vi "Execute.vi"(0 "Session Handle in":T4, 1 "Sequence Name":string, 5 "SequenceFile":T3, 9 "Parameters (None)":T2, 11 "error in (no error)":errorcluster, 12 "ProcessModel (None)":T3) -> (4 "Session Handle out":T4, 10 "Execution":T1, 15 "error out":errorcluster)   [LabVIEW 2019, in "HTS.lvlib" / "Engine.lvclass"]
uses:
  Engine.lvclass
  Typedefs/Session Handle.ctl
  SequenceFile/SequenceFile.lvclass
  SequenceFile/Typedefs/Session Handle.ctl
  VariableContainer/VariableContainer.lvclass
  VariableContainer/Typedefs/Session Handle.ctl
  Execution/Execution.lvclass
  Execution/Typedefs/Session Handle.ctl
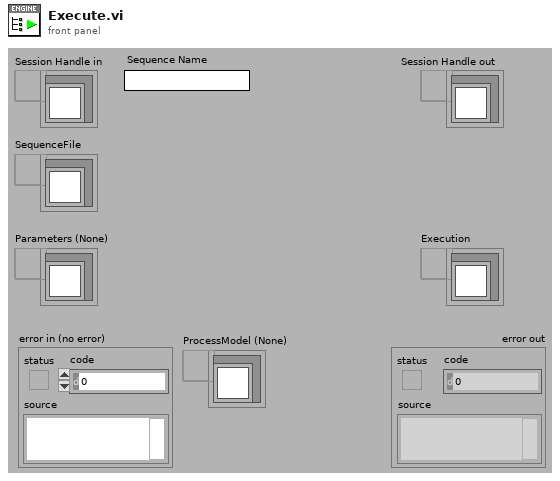
[diagram p1: front panel]
types:
  T1 = typedef "HTS.lvlib/Execution.lvclass/Session Handle.ctl" = refnum<data-value>
  T2 = typedef "HTS.lvlib/VariableContainer.lvclass/Session Handle.ctl" = refnum<data-value>
  T3 = typedef "HTS.lvlib/SequenceFile.lvclass/Session Handle.ctl" = refnum<data-value>
  T4 = typedef "HTS.lvlib/Engine.lvclass/Session Handle.ctl" = refnum<data-value>
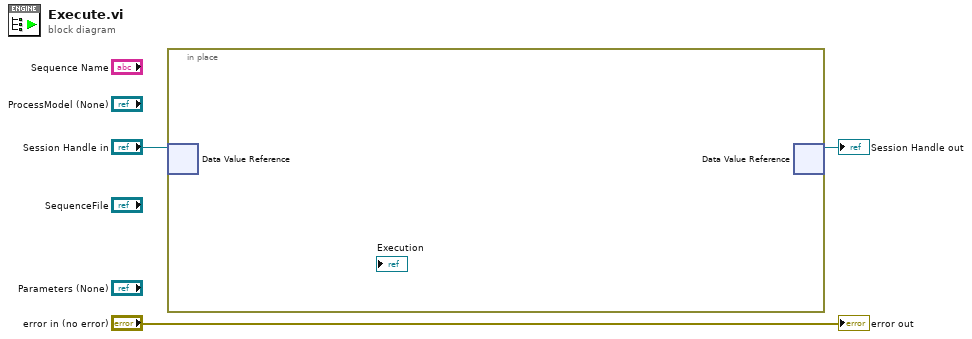
[diagram p0: block diagram]
diagram:
  n1 = in-place {
    n2 = in-place-dvr #1("Session Handle in") -> ()  [unwired: 2 out]
    n3 = in-place-dvr #1() -> (→"Session Handle out":T4)  [unwired: 1 in, 1 out]
  }
  "error out" <- "error in (no error)"
